vi "VisionControl.vi"() -> (2 "Right Drive":dbl, 3 "Left Drive":dbl)   [LabVIEW 2015]
uses:
  Utilities/GlobalVisionVars.vi
  <vilib>/addons/control/pid/pid.llb/PID (DBL).vi
  <vilib>/addons/control/pid/NI_PID_pid.lvlib
  navx-mxp/labview/navX Library v2/navX Library v2.lvlib
panel:
  in  "upper limit3":dbl=0.18 format="%#_13g"
  in  "PID gains 2":T1={"proportional gain (Kc)"=50.0, "integral time (Ti, min)"=0.0, "derivative time (Td, min)"=0.0015} {"derivative time (Td, min)" format="%.5f"; "integral time (Ti, min)" format="%.3f"; "proportional gain (Kc)" format="%.3f"}
  in  "y":dbl=8.0
  in  "upper limit2":dbl=0.24 format="%#_13g"
  in  "upper limit1":dbl=0.4 format="%#_13g"
  out "DesiredGyroValue":dbl
  out "Angle":dbl
  in  "PID gains":T1={"proportional gain (Kc)"=20.0, "integral time (Ti, min)"=0.0, "derivative time (Td, min)"=0.0015} {"derivative time (Td, min)" format="%.5f"; "integral time (Ti, min)" format="%.3f"; "proportional gain (Kc)" format="%.3f"}
  in  "error in (no error)":errorcluster
  # "22"
  # "0.3\n0.3"
  # "CompBot"
  # "PracticeBot"
  # "New"
  # "P=12"
  # "P=10.8"
  # "P=20"
  # "D=0.00150"
  # "D=0"
  # "D=0.00150"
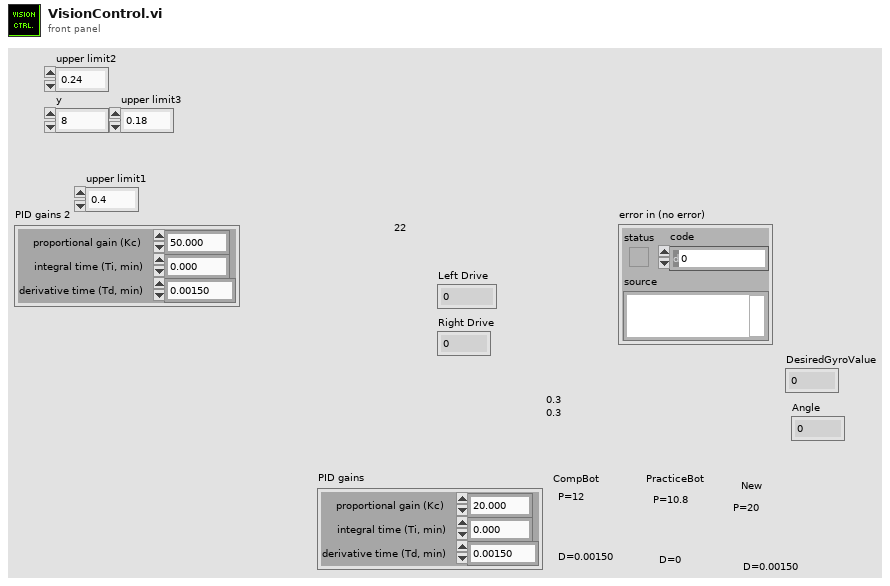
[diagram p1: front panel]
types:
  T1 = cluster{"proportional gain (Kc)":dbl, "integral time (Ti, min)":dbl, "derivative time (Td, min)":dbl}
  T2 = typedef "navX Library v2.lvlib/Z900_navX_DeviceTypeDef.ctl" = cluster{"Interface":cluster{"Protocol":T3, "Update Rate (4Hz-60Hz)":u8, "navX Open TypeDef":variant}, "Notify Packet":refnum<notifier>, "Loop VI Refnum":refnum<vi>, "Ready to Close Occurrence Refnum":refnum<k4>}
  T3 = typedef "navX Library v2.lvlib/Z900_navX_ProtocolTypeDef.ctl" = enum16{"SERIAL", "I2C", "SPI"}
  T4 = cluster{"Yaw":dbl, "Roll":dbl, "Pitch":dbl, "Heading":dbl, "Fused Heading":dbl}
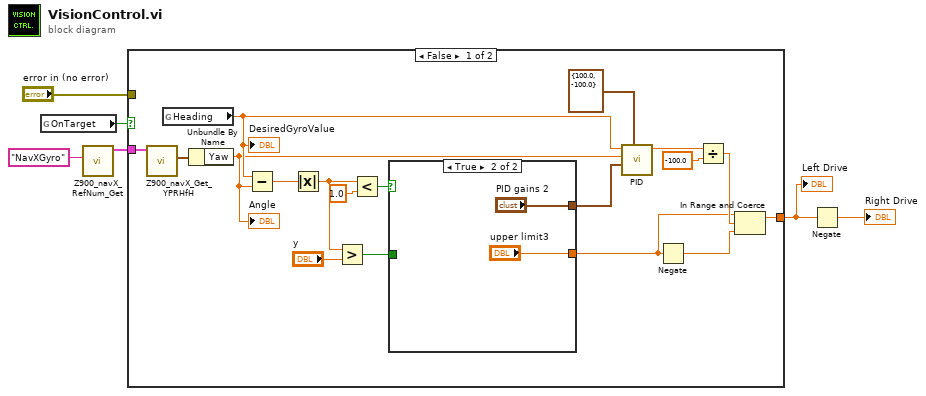
[diagram p0: block diagram]
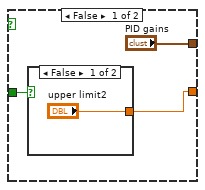
[diagram p2: hidden frame]
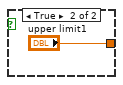
[diagram p3: hidden frame]
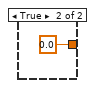
[diagram p4: hidden frame]
diagram:
  n1 = global read "GlobalVisionVars.vi" "OnTarget"() -> (w3:bool)
  n2 = call "Z900_navX_RefNum_Get.vi"("refnum name"="NavXGyro") -> ("navX Device"=w1:T2)  [unwired: 9 in, 1 out]
  n3 = case shown="False" w3 {
    tunnel: [w20 0.0 ("upper limit")] -> w4
    tunnel: "error in (no error)" -> [_ _]
    tunnel: w1 -> [w16 _]
    frame False {
      n4 = call "Z900_navX_Get_YPRHfH.vi"("navX Device"=w16) -> ("YRPHfH"=w17:T4)  [unwired: 7 in, 3 out]
      n5 = global read "GlobalVisionVars.vi" "Heading"() -> (w15:dbl)
      "DesiredGyroValue" <- w15
      n6 = Unbundle By Name(w17) -> ("Yaw"=w14:dbl)
      "Angle" <- w14
      n7 = Subtract(x=w15, y=w14) -> (x-y=w13:dbl)
      n8 = Absolute Value(x=w13) -> (abs(x)=w10:dbl)
      n9 = Greater?(x=w10, y="y") -> (0:w12:bool)
      n10 = Less?(x=w10, y=1.0) -> (x < y?=w8:bool)
      n11 = case shown="True" w8 {
        tunnel: [w27 "upper limit3"] -> w19
        tunnel: w12 -> [w26 _]
        tunnel: ["PID gains" "PID gains 2"] -> w7
        frame False {
          n12 = case shown="False" w26 {
            tunnel: ["upper limit2" "upper limit1"] -> w27
            frame False {
            }
            frame True {
            }
          }
        }
        frame True {
        }
      }
      n13 = call-poly <vilib>:"PID.vi"("output range"=cluster{"output high":dbl, "output low":dbl} {"output high"=100.0, "output low"=-100.0}, "PID gains"=w7, "process variable"=w14, "setpoint"=w15) -> ("output"=w23:dbl)  [unwired: 6 in, 1 out]
      n14 = Negate(x=w19) -> (-x=w18:dbl)
      n15 = Divide(x=w23, y=-100.0) -> (x/y=w21:dbl)
      n16 = In Range and Coerce(upper limit=w19, x=w21, lower limit=w18) -> (coerced(x)=w20:dbl)  [unwired: 1 out]
    }
    frame True {
    }
  }
  "Left Drive" <- w4
  n17 = Negate(x=w4) -> (-x=→"Right Drive":dbl)
